vi "MapScriptActor.vi"(8 "error in (no error)":errorcluster) -> (0 "error out":errorcluster)   [LabVIEW 2017]
doc: "Use this template to build a VI to use as a subVI."
uses:
  MapScriptMeasurementStateMachineEnum.ctl
  Spectrometer Utilities/SpectrometerControllerEnum.ctl
  Spectrometer Utilities/SpectrometerCallbackdataEvent.ctl
  Microscope/MicroscopeControllerCluster.ctl
  <vilib>/vision/Image Controls.llb/IMAQ Image.ctl
  Microscope/MicroscopeControllerEnum.ctl
  Database/DatabaseContollerGFVenum.ctl
  MapScriptGFVEnum.ctl
  Spectrometer Utilities/SpectrometerData.ctl
  AEROTECstageAPI/StageEnum.ctl
  MapScriptDataGFV.ctl
  SpectroMeasurementCtrlEnum.ctl
panel:
  in  "Reset Measurement":bool
  in  "CaptureMicroscopeImageButton":bool
  out "User Picture":T1(plugin-control)
  in  "Add/Remove User 2":bool
  in  "Sample Type":u16(ring) caption="Combo Box" items=["Solid", "Liquid"]
  out "Experiment No.":i32 caption="String"
  in  "Experiment Title":string caption="String"
  out "Measurement State":T2
  out "Measurement points left in queue":i32
  out "Number of Points Selected":i32
  in  "abort":bool
  out "Measurement\nCompleted\nSuccessfully":bool
  out "Measurement\nIn\nProgress":bool
  in  "Stop":bool
  in  "Run":bool
  # "Map script"
  # "Total Measurment Time Estimate"
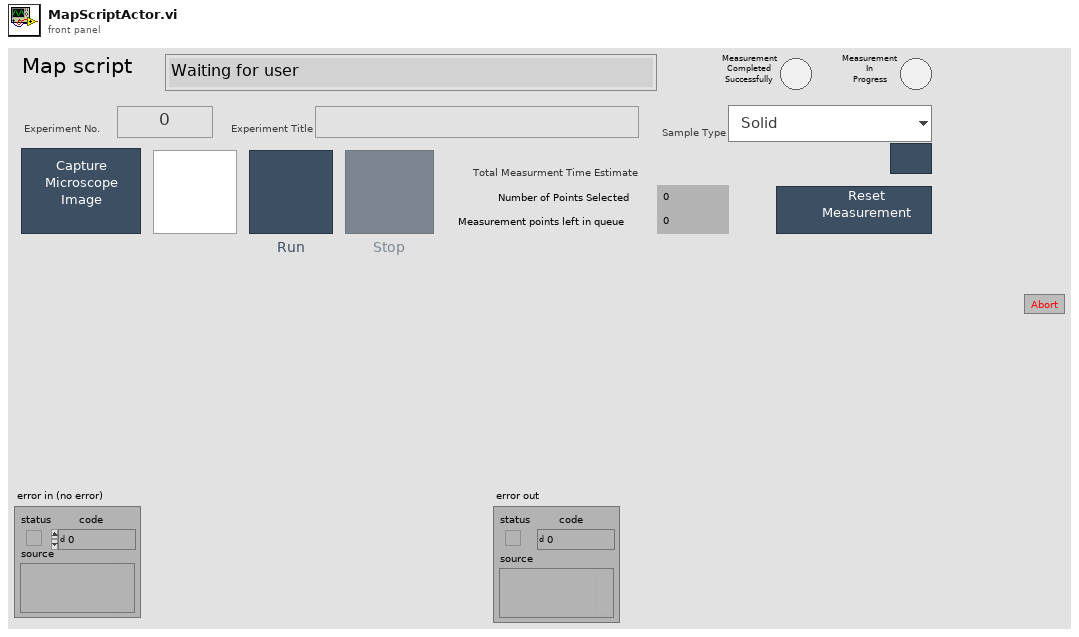
[diagram p1: front panel]
types:
  T1 = typedef "IMAQ Image.ctl" = refnum<image>
  T2 = typedef "MapScriptMeasurementStateMachineEnum.ctl" = enum16{"Waiting for user", "Moving the stage", "Verifying stage moved Successfully", "Running Raman measurement", "Waiting for measurement to finish", "Updating database with results"}
  T3 = typedef "MapScriptGFVEnum.ctl" = enum16{"GetAllData!", "InsertCoordData!", "InsertExperimentTitle", "Init!", "Stop!", "Start!", "GetMapScriptActorViRef", "InsertExperimentNumber", "InsertSampleType", "InsertMicroscopeImage"}
  T4 = typedef "DatabaseContollerGFVenum.ctl" = enum16{"Init and Open Database!", "GetNewMeas_dataIndex", "UpdateWithSpectrometerData", "UpdateWithMicroscopeData", "UpdateWithMapScriptData", "UpdateWithmainUIData", "Get Objective Microns/Pixels", "Get User Name!", "Get Active Users Names!", "Get User Picture!", "Get User Phone Number!", "Get Setup Names!", "Get Active Microscope Objectives!", "Get Experiment Number!", "Get Sample Types!", "Write meas_conf Table", "Write meas_data Table", "GetListOfIndices", "Get Objective Index"}
  T5 = cluster{"Stop":bool, "Point":cluster{"X":sgl, "Y":sgl}, "PointIndex":i32}
  T6 = typedef "MicroscopeControllerEnum.ctl" = enum16{"GetAllData!", "Init!", "Start!", "Stop!", "GetMicroscopeVIRef", "CalculateRelPointForStagemicrons", "InsertCallbackEvent!", "InsertLaserPoint!", "InsertMapPoints!", "InsertMicroscopeImageRef!", "GetMicroscopeImageRef", "InsertObjectiveIndex!"}
  T7 = typedef "SpectrometerControllerEnum.ctl" = enum16{"Init!", "Start!", "Stop!", "Start New Measurement!", "Update Current Measurement Data", "Set Current Measurement Ended Successfully", "Get Current Measurement Data!", "Get Current Measurement Ended Successfully", "GetSpectrometerVIRef!", "Insert Callback Event", "GetAllData!"}
  T8 = typedef "StageEnum.ctl" = enum16{"Get Current Pos!", "Move axis!", "Enable Stage!", "Stop Stage Controller!", "Set Default Speeds!", "Get Stage Parameters", "Start Stage Controller!", "Init", "Go Home!"}
  T9 = typedef "MapScriptDataGFV.ctl" = cluster{"idMeasConf":u32, "ExperimentTitle":string, "idsample_type":u32, "MicroscopeImage":string, "MeasPointNum":u32, "XCoorRequestedPixel":u32, "YCoorRequestedPixel":u32, "XCoorRequestedMicrons":dbl, "YCoorRequestedMicrons":dbl, "XCoorMeasuredMicrons":dbl, "YCoorMeasuredMicrons":dbl, "idMeasData":u32}
  T10 = typedef "MicroscopeControllerCluster.ctl" = cluster{"MapPointsArray":cluster{"X":i32, "Y":i32}[], "Laser Point Coor":cluster{"X":i32, "Y":i32}, "Microscope Image Ref":T1, "idObjectives":u32}
  T11 = typedef "SpectroMeasurementCtrlEnum.ctl" = enum16{"Init", "InsertMeasurementScript", "InsertSetupIndex", "InsertCurrentUserIndex", "GetAllData!"}
  T12 = typedef "SpectrometerData.ctl" = cluster{"Acquisition Time":dbl, "Range Begin":dbl, "Acquistion Time Unit":string, "Accumulations":i32, "Range End":dbl, "Range Unit":string, "Windows":i32, "Auto Focus":bool, "Auto Exposure":bool, "Spike Filter":string, "Delay Time":dbl, "Delay Time Unit":string, "Binning":i32, "Readout Mode":string, "DeNoise":bool, "ICS correction":bool, "Dark correction":bool, "Instrument Process":bool, "Instrument":string, "Detector":string, "Objective":string, "Grating":i32, "Grating Unit":string, "ND Filter":dbl, "ND Filter Unit":string, "Laser":dbl, "Laser Unit":string, "Slit":dbl, "Hole":dbl, "Acquired DateTime":string, "X axis":dbl[], "Y axis":dbl[]}
  T13 = enum8{"Enabled", "Disabled", "Disabled and Grayed Out"}
  T14 = typedef "SpectrometerCallbackdataEvent.ctl" = cluster{"MeasurementEndedSuccessfully?":bool, "Spectrometer Connected?":bool, "Measurement In Progress?":bool}
  T15 = typedef "Image Type" = u32
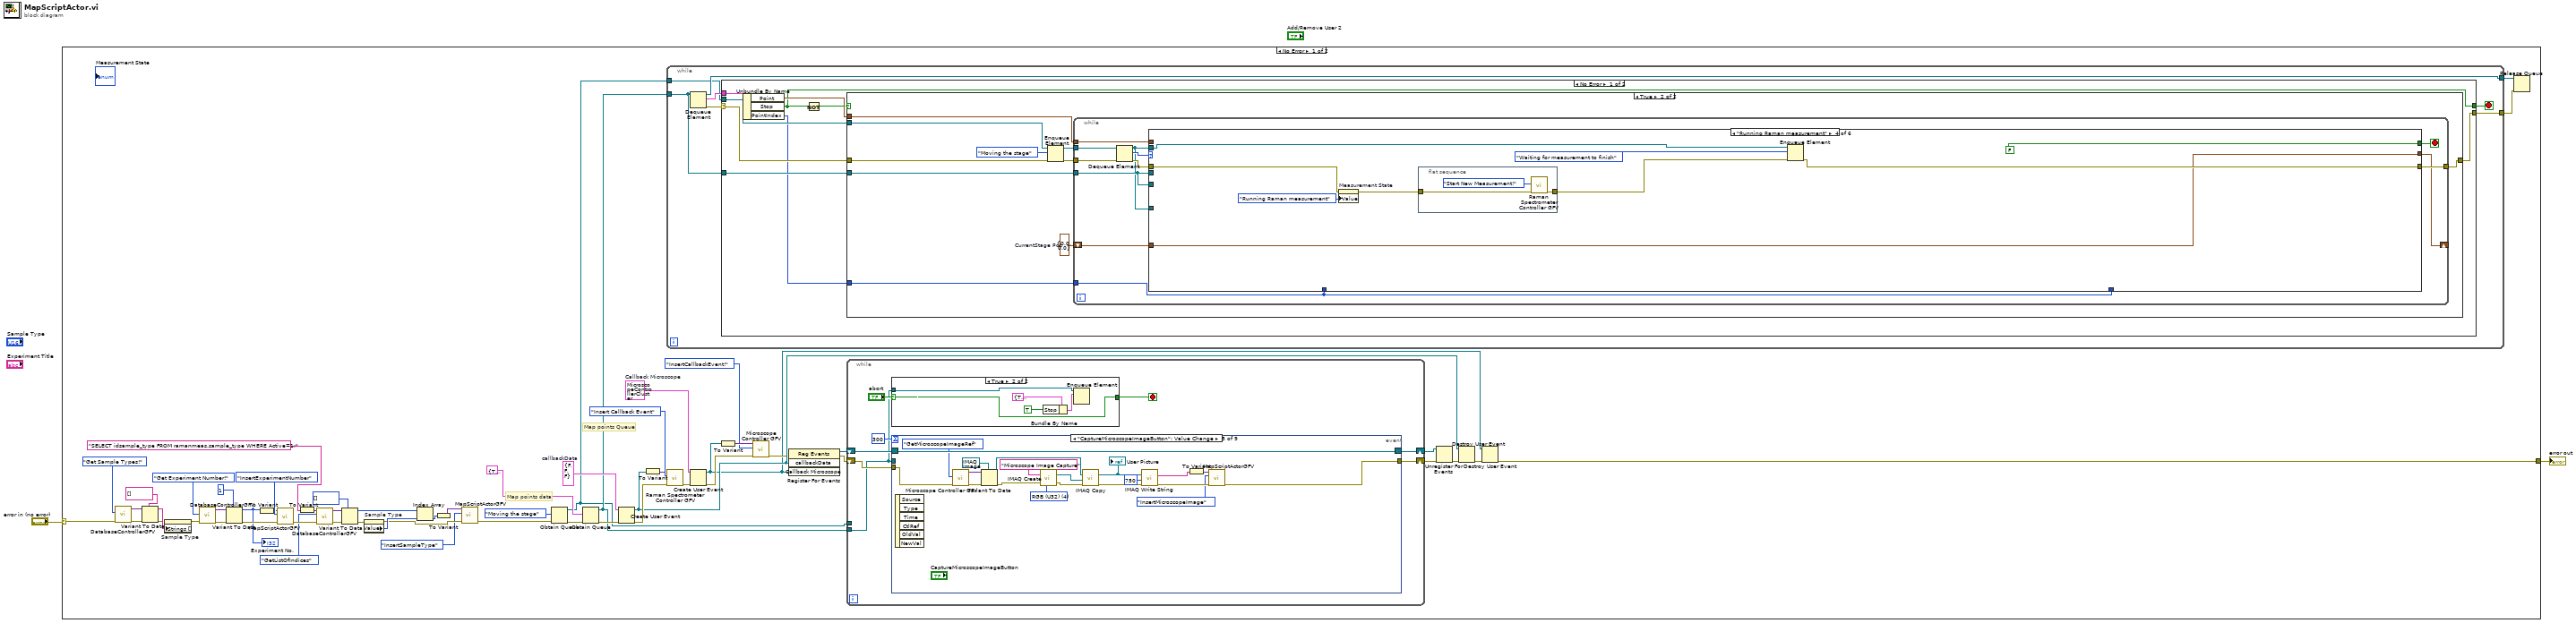
[diagram p0: block diagram]
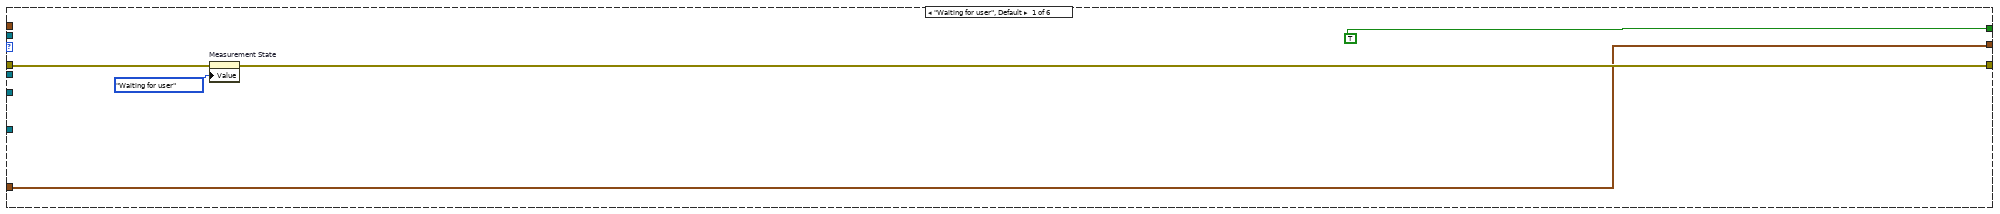
[diagram p3: hidden frame]
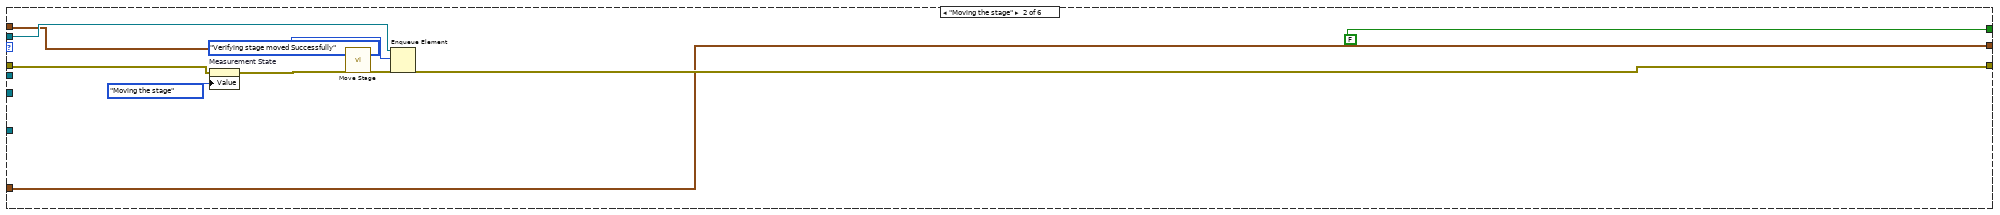
[diagram p4: hidden frame]
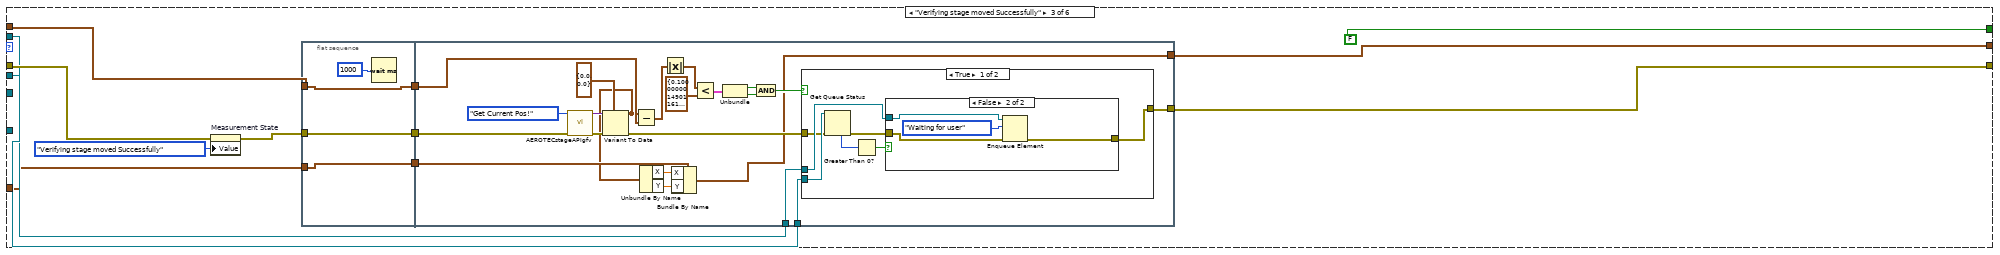
[diagram p5: hidden frame]
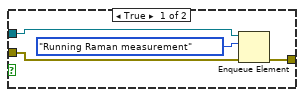
[diagram p6: hidden frame]
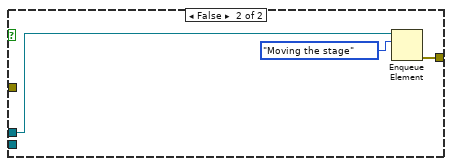
[diagram p7: hidden frame]
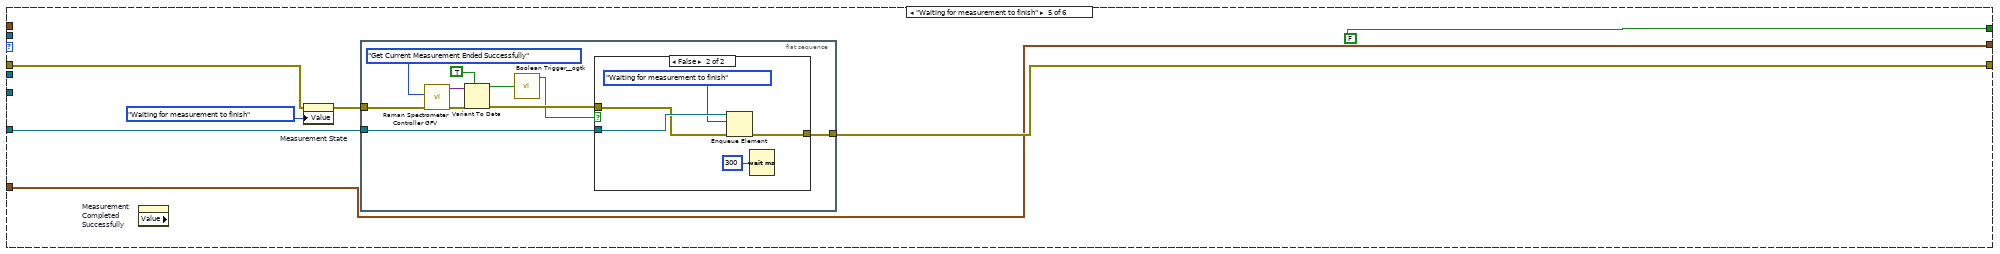
[diagram p8: hidden frame]
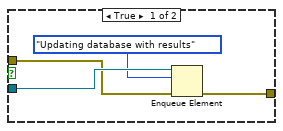
[diagram p9: hidden frame]
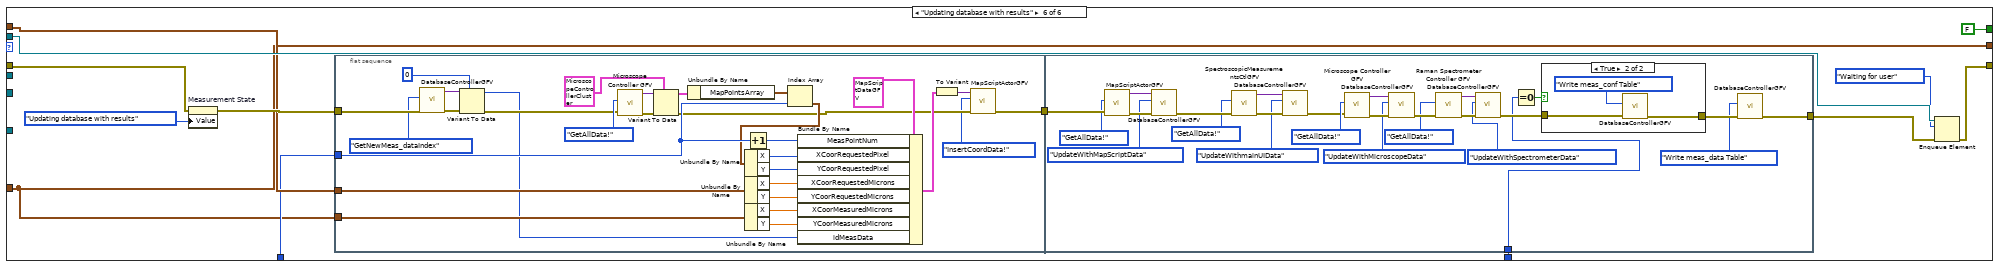
[diagram p10: hidden frame]
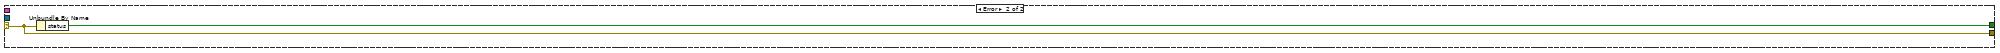
[diagram p12: hidden frame]
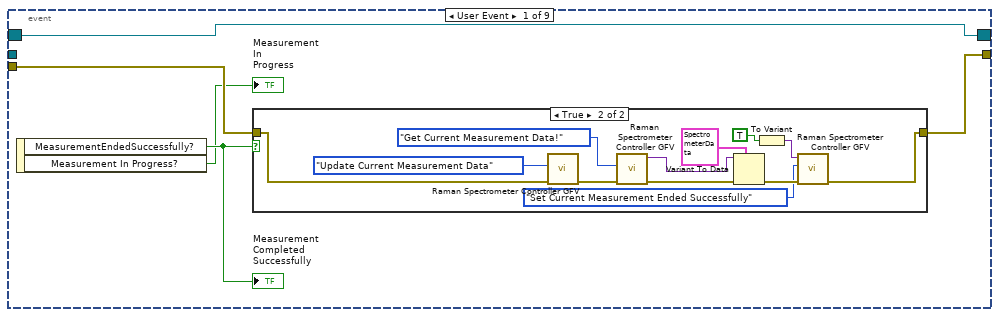
[diagram p14: hidden frame]
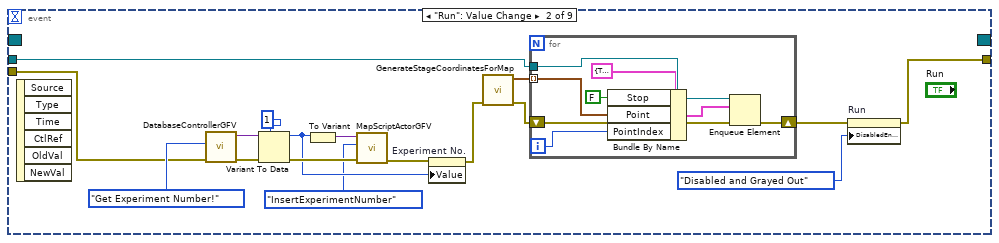
[diagram p16: hidden frame]
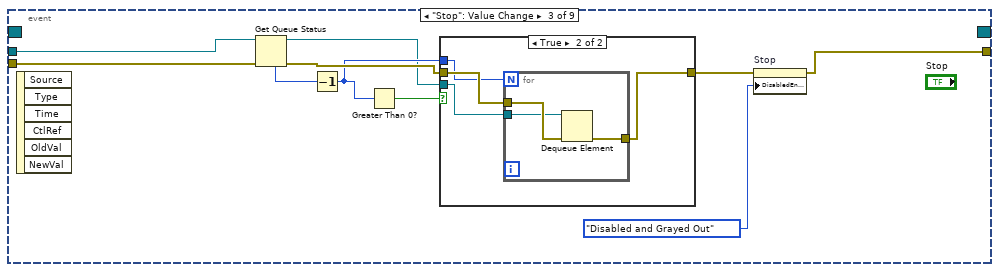
[diagram p17: hidden frame]
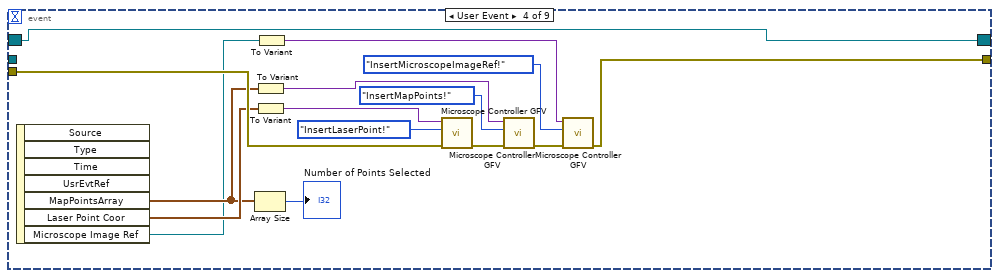
[diagram p19: hidden frame]
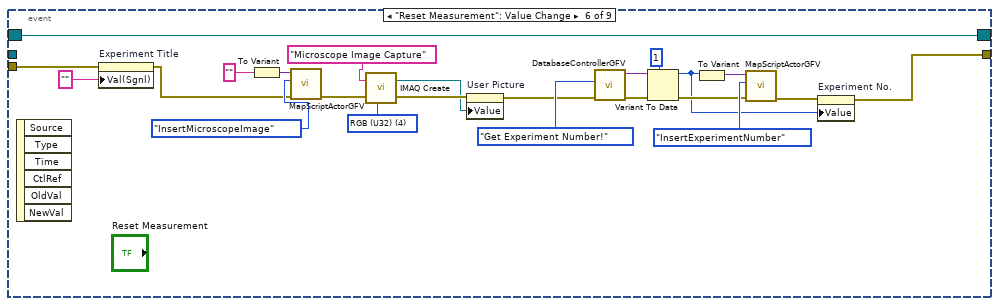
[diagram p20: hidden frame]
diagram:
  n1 = case shown="No Error" "error in (no error)" {
    selector: "error in (no error)" -> [w22 w456]
    tunnel: [w38 w456] -> w1
    frame No Error {
      w50 = T10 {"MapPointsArray"=[], "Laser Point Coor"={"X"=0, "Y"=0}, "Microscope Image Ref"=refnum, "idObjectives"=0}  # Callback Microscope
      w59 = T14 {"MeasurementEndedSuccessfully?"=FALSE, "Spectrometer Connected?"=FALSE, "Measurement In Progress?"=FALSE}  # callbackData
      # "Map points data"
      # "Map points Queue"
      n2 = call "DatabaseControllerGFV.vi"("error in (no error)"=w22, "Enum"=DatabaseContollerGFVenum."Get Sample Types!") -> ("error out"=w29:errorcluster, "Data Out"=w28:variant)  [unwired: 8 in]
      n3 = Variant To Data(error in=w29, type=string[] [] ("Strings []"), Variant=w28) -> (data=w25:string[], error out=w23:errorcluster)
      n4 = property on="Sample Type" class="Ring (strict)"(error in=w23, "Strings []"=w25) -> (error out=w24:errorcluster)  [unwired: 1 in, 1 out]
      n5 = call "DatabaseControllerGFV.vi"("error in (no error)"=w24, "Enum"=DatabaseContollerGFVenum."Get Experiment Number!") -> ("error out"=w31:errorcluster, "Data Out"=w32:variant)  [unwired: 8 in]
      n6 = Variant To Data(error in=w31, type=1, Variant=w32) -> (data=w18:i32, error out=w21:errorcluster)
      "Experiment No." <- w18
      n7 = To Variant(anything=w18) -> (Variant=w19:variant)
      n8 = call "MapScriptActorGFV.vi"("error in (no error)"=w21, "MapScriptEnum"=MapScriptGFVEnum."InsertExperimentNumber", "Data in"=w19) -> ("error out"=w17:errorcluster)  [unwired: 7 in, 1 out]
      n9 = To Variant(anything="SELECT idsample_type FROM ramanmeas.sample_type WHERE Active=1;") -> (Variant=w16:variant)
      n10 = call "DatabaseControllerGFV.vi"("error in (no error)"=w17, "Enum"=DatabaseContollerGFVenum."GetListOfIndices", "Data in"=w16) -> ("error out"=w13:errorcluster, "Data Out"=w12:variant)  [unwired: 7 in]
      n11 = Variant To Data(error in=w13, type=i32[] [], Variant=w12) -> (data=w10:i32[], error out=w9:errorcluster)
      n12 = property on="Sample Type" class="Ring (strict)"(error in=w9) -> (error out=w7:errorcluster, "Value"=w8:u16)  [unwired: 1 in, 1 out]
      n13 = Index Array(array=w10, index=w8) -> (element=w4:i32)
      n14 = To Variant(anything=w4) -> (Variant=w3:variant)
      n15 = call "MapScriptActorGFV.vi"("error in (no error)"=w7, "MapScriptEnum"=MapScriptGFVEnum."InsertSampleType", "Data in"=w3) -> ("error out"=w6:errorcluster)  [unwired: 7 in, 1 out]
      n16 = Obtain Queue(element data type=MapScriptMeasurementStateMachineEnum."Moving the stage" ("element"), error in (no error)=w6) -> (queue out=w35:refnum<queue>, error out=w36:errorcluster)  [unwired: 3 in, 1 out]
      n17 = Obtain Queue(element data type=T5 {"Stop"=TRUE, "Point"={"X"=0.0, "Y"=0.0}, "PointIndex"=0}, error in (no error)=w36) -> (queue out=w41:refnum<queue>, error out=w42:errorcluster)  [unwired: 3 in, 1 out]
      n18 = Create User Event(user event datatype=w59, error in=w42) -> (user event=w52:refnum<user-event>, error out=w58:errorcluster)
      n19 = To Variant(anything=w52) -> (Variant=w57:variant)
      n20 = while {
        tunnel: w41 -> [w61]
        tunnel: [w65] -> w40
        tunnel: [w64] -> w39
        tunnel: w35 -> [w62]
        stop <- w63 stop-if-true
        n21 = Dequeue Element(queue=w61) -> (queue out=w65:refnum<queue>, element=w66:T5, error out=w67:errorcluster)  [unwired: 2 in, 1 out]
        n22 = case shown="No Error" w67 {
          selector: w67 -> [w72 w284]
          tunnel: w66 -> [w76 _]
          tunnel: [w71 w284] -> w64
          tunnel: [w73 w283] -> w63
          tunnel: w62 -> [w70 _]
          tunnel: w61 -> [w69 _]
          frame No Error {
            n23 = Unbundle By Name(w76) -> ("Point"=w75:cluster{"X":sgl, "Y":sgl}, "Stop"=w73:bool, "PointIndex"=w68:i32)
            n24 = Not(x=w73) -> (.not. x?=w74:bool)
            n25 = case shown="True" w74 {
              tunnel: w75 -> [_ w87]
              tunnel: w72 -> [w77 w84]
              tunnel: [w77 w82] -> w71
              tunnel: w70 -> [_ w86]
              tunnel: w69 -> [_ w80]
              tunnel: w68 -> [_ w78]
              frame False {
              }
              frame True {
                w79 = cluster{"X":sgl, "Y":sgl} {"X"=0.0, "Y"=0.0}  # CurrentStage Pos
                n26 = Enqueue Element(queue=w86, element=MapScriptMeasurementStateMachineEnum."Moving the stage", error in (no error)=w84) -> (queue out=w85:refnum<queue>, error out=w83:errorcluster)  [unwired: 1 in, 1 out]
                n27 = while {
                  tunnel: w85 -> [w99]
                  tunnel: w83 -> [w98]
                  tunnel: w87 -> [w95]
                  tunnel: [w91] -> w82
                  tunnel: w80 -> [w93]
                  shift-right: [w90] -> _
                  shift-left: w79 -> [w88]
                  tunnel: w78 -> [w89]
                  stop <- w96 stop-if-true
                  n28 = Dequeue Element(queue=w99, error in (no error)=w98) -> (queue out=w92:refnum<queue>, element=w94:T2, error out=w97:errorcluster)  [unwired: 1 in, 1 out]
                  n29 = case shown="\"Running Raman measurement\"" w94 {
                    tunnel: w97 -> [w102 w113 w126 w179 w190 w221]
                    tunnel: [TRUE FALSE FALSE FALSE FALSE FALSE] -> w96
                    tunnel: w95 -> [_ w108 w123 _ _ w213]
                    tunnel: w92 -> [_ w112 w120 w177 _ w218]
                    tunnel: w93 -> [_ _ _ _ _ _]
                    tunnel: w93 -> [_ _ w122 _ _ _]
                    tunnel: [w101 w106 w121 w175 w186 w215] -> w91
                    tunnel: w92 -> [_ _ _ _ w187 _]
                    tunnel: [w100 w105 w117 w172 w184 w211] -> w90
                    tunnel: w88 -> [w100 w105 w116 w172 w184 w211]
                    tunnel: w89 -> [_ _ _ _ _ w212]
                    tunnel: w89 -> [_ _ _ _ _ w210]
                    frame "Waiting for user", Default {
                      n30 = property on="Measurement State" class="Enum (strict)"(error in=w102, "Value"=MapScriptMeasurementStateMachineEnum."Waiting for user" ("element")) -> (error out=w101:errorcluster)  [unwired: 1 in, 1 out]
                    }
                    frame "Moving the stage" {
                      n31 = property on="Measurement State" class="Enum (strict)"(error in=w113, "Value"=MapScriptMeasurementStateMachineEnum."Moving the stage" ("element")) -> (error out=w109:errorcluster)  [unwired: 1 in, 1 out]
                      n32 = call "Move Stage.vi"("error in (no error)"=w109, "Input Coor"=w108) -> ("error out"=w107:errorcluster)  [unwired: 9 in]
                      n33 = Enqueue Element(queue=w112, element=MapScriptMeasurementStateMachineEnum."Verifying stage moved Successfully", error in (no error)=w107) -> (error out=w106:errorcluster)  [unwired: 1 in, 2 out]
                    }
                    frame "Verifying stage moved Successfully" {
                      n34 = property on="Measurement State" class="Enum (strict)"(error in=w126, "Value"=MapScriptMeasurementStateMachineEnum."Verifying stage moved Successfully" ("element")) -> (error out=w125:errorcluster)  [unwired: 1 in, 1 out]
                      n35 = flat-sequence {
                        tunnel: w123 -> [w130]
                        tunnel: w125 -> [w131]
                        tunnel: [w131] -> w119
                        tunnel: [w130] -> w118
                        tunnel: w116 -> [w128]
                        tunnel: [w128] -> w115
                        tunnel: w120 -> [w140]
                        tunnel: w122 -> [w139]
                        tunnel: [w138] -> w121
                        tunnel: w119 -> [w149]
                        tunnel: w118 -> [w148]
                        tunnel: [w135] -> w117
                        tunnel: w115 -> [w136]
                        frame #0 {
                          n36 = Wait (ms)(milliseconds to wait=u32 1000) -> ()  [unwired: 1 out]
                        }
                        frame #1 {
                          n37 = call "AEROTECstageAPIgfv.vi"("error in (no error)"=w149, "StageContrlEnum"=StageEnum."Get Current Pos!") -> ("error out"=w150:errorcluster, "Data Out"=w152:variant)  [unwired: 8 in]
                          n38 = Variant To Data(error in=w150, type=cluster{"X":sgl, "Y":sgl} {"X"=0.0, "Y"=0.0}, Variant=w152) -> (data=w134:cluster{"X":sgl, "Y":sgl}, error out=w137:errorcluster)
                          n39 = Subtract(x=w134, y=w148) -> (x-y=w147:cluster{"X":sgl, "Y":sgl})
                          n40 = Unbundle By Name(w134) -> ("X"=w133:sgl, "Y"=w132:sgl)
                          n41 = Absolute Value(x=w147) -> (abs(x)=w146:cluster{"X":sgl, "Y":sgl})
                          n42 = Bundle By Name(cluster=w136, "X"=w133, "Y"=w132) -> (w135:cluster{"X":sgl, "Y":sgl})
                          n43 = Less?(x=w146, y=cluster{"X":sgl, "Y":sgl} {"X"=0.1, "Y"=0.1}) -> (x < y?=w144:cluster{"X":bool, "Y":bool})
                          n44 = Unbundle(w144) -> ("X"=w143:bool, "Y"=w142:bool)
                          n45 = And(x=w143, y=w142) -> (x .and. y?=w141:bool)
                          n46 = case shown="True" w141 {
                            tunnel: w140 -> [w157 w171]
                            tunnel: w139 -> [w156 _]
                            tunnel: [w155 w170] -> w138
                            tunnel: w137 -> [w154 _]
                            frame True {
                              n47 = Get Queue Status(queue=w156, error in (no error)=w154) -> (error out=w158:errorcluster, # elements in queue=w159:i32)  [unwired: 1 in, 6 out]
                              n48 = Greater Than 0?(x=w159) -> (x > 0?=w160:bool)
                              n49 = case shown="False" w160 {
                                tunnel: [w164 w168] -> w155
                                tunnel: w157 -> [w163 w167]
                                tunnel: w158 -> [w161 w165]
                                frame True {
                                n50 = Enqueue Element(queue=w163, element=MapScriptMeasurementStateMachineEnum."Running Raman measurement", error in (no error)=w161) -> (error out=w164:errorcluster)  [unwired: 1 in, 2 out]
                                }
                                frame False {
                                n51 = Enqueue Element(queue=w167, element=MapScriptMeasurementStateMachineEnum."Waiting for user", error in (no error)=w165) -> (error out=w168:errorcluster)  [unwired: 1 in, 2 out]
                                }
                              }
                            }
                            frame False {
                              n52 = Enqueue Element(queue=w171, element=MapScriptMeasurementStateMachineEnum."Moving the stage") -> (error out=w170:errorcluster)  [unwired: 2 in, 2 out]
                            }
                          }
                        }
                      }
                    }
                    frame "Running Raman measurement" {
                      n53 = property on="Measurement State" class="Enum (strict)"(error in=w179, "Value"=MapScriptMeasurementStateMachineEnum."Running Raman measurement" ("element")) -> (error out=w178:errorcluster)  [unwired: 1 in, 1 out]
                      n54 = flat-sequence {
                        tunnel: w178 -> [w182]
                        tunnel: [w181] -> w174
                        frame #0 {
                          n55 = call "Raman Spectrometer Controller GFV.vi"("SpectrometerEnum"=SpectrometerControllerEnum."Start New Measurement!", "error in (no error)"=w182) -> ("error out"=w181:errorcluster)  [unwired: 7 in, 1 out]
                        }
                      }
                      n56 = Enqueue Element(queue=w177, element=MapScriptMeasurementStateMachineEnum."Waiting for measurement to finish", error in (no error)=w174) -> (error out=w175:errorcluster)  [unwired: 1 in, 2 out]
                    }
                    frame "Waiting for measurement to finish" {
                      n57 = property on="Measurement\nCompleted\nSuccessfully" class="Bool (strict)" props=["Value"]() -> ()  [unwired: 2 in, 3 out]
                      n58 = property on="Measurement State" class="Enum (strict)"(error in=w190, "Value"=MapScriptMeasurementStateMachineEnum."Waiting for measurement to finish" ("element")) -> (error out=w189:errorcluster)  [unwired: 1 in, 1 out]
                      n59 = flat-sequence {
                        tunnel: w189 -> [w198]
                        tunnel: w187 -> [w200]
                        tunnel: [w199] -> w186
                        frame #0 {
                          n60 = call "Raman Spectrometer Controller GFV.vi"("SpectrometerEnum"=SpectrometerControllerEnum."Get Current Measurement Ended Successfully", "error in (no error)"=w198) -> ("Data Out"=w195:variant, "error out"=w196:errorcluster)  [unwired: 7 in]
                          n61 = Variant To Data(error in=w196, type=TRUE, Variant=w195) -> (data=w192:bool, error out=w193:errorcluster)
                          n62 = call <userlib>:"Boolean Trigger__ogtk.vi"("Boolean Input"=w192) -> ("Rising Edge"=w191:bool)  [unwired: 1 in, 1 out]
                          n63 = case shown="False" w191 {
                            tunnel: w200 -> [w204 w209]
                            tunnel: [w203 w208] -> w199
                            tunnel: w193 -> [w201 w206]
                            frame True {
                              n64 = Enqueue Element(queue=w204, element=MapScriptMeasurementStateMachineEnum."Updating database with results", error in (no error)=w201) -> (error out=w203:errorcluster)  [unwired: 1 in, 2 out]
                            }
                            frame False {
                              n65 = Enqueue Element(queue=w209, element=MapScriptMeasurementStateMachineEnum."Waiting for measurement to finish", error in (no error)=w206) -> (error out=w208:errorcluster)  [unwired: 1 in, 2 out]
                              n66 = Wait (ms)(milliseconds to wait=u32 300) -> ()  [unwired: 1 out]
                            }
                          }
                        }
                      }
                    }
                    frame "Updating database with results" {
                      n67 = property on="Measurement State" class="Enum (strict)"(error in=w221, "Value"=MapScriptMeasurementStateMachineEnum."Updating database with results" ("element")) -> (error out=w220:errorcluster)  [unwired: 1 in, 1 out]
                      n68 = flat-sequence {
                        tunnel: w220 -> [w229]
                        tunnel: [w231] -> w214
                        tunnel: w213 -> [w240]
                        tunnel: w211 -> [w243]
                        tunnel: w212 -> [w244]
                        tunnel: [w254] -> w219
                        tunnel: w214 -> [w278]
                        tunnel: w210 -> [w256]
                        frame #0 {
                          n69 = call "DatabaseControllerGFV.vi"("error in (no error)"=w229, "Enum"=DatabaseContollerGFVenum."GetNewMeas_dataIndex") -> ("error out"=w228:errorcluster, "Data Out"=w225:variant)  [unwired: 8 in]
                          n70 = Variant To Data(error in=w228, type=0, Variant=w225) -> (data=w223:i32, error out=w227:errorcluster)
                          n71 = call "Microscope Controller GFV.vi"("error in (no error)"=w227, "MicroscopeEnum"=MicroscopeControllerEnum."GetAllData!") -> ("error out"=w251:errorcluster, "Data Out"=w250:variant)  [unwired: 8 in]
                          n72 = Variant To Data(error in=w251, type=T10 {"MapPointsArray"=[], "Laser Point Coor"={"X"=0, "Y"=0}, "Microscope Image Ref"=refnum, "idObjectives"=0}, Variant=w250) -> (data=w248:T10, error out=w232:errorcluster)
                          n73 = Unbundle By Name(w248) -> ("MapPointsArray"=w247:cluster{"X":i32, "Y":i32}[])
                          n74 = Unbundle By Name(w240) -> ("X"=w239:sgl, "Y"=w238:sgl)
                          n75 = Unbundle By Name(w243) -> ("X"=w242:sgl, "Y"=w241:sgl)
                          n76 = Increment(x=w244) -> (x+1=w245:i32)
                          n77 = Index Array(array=w247, index=w244) -> (element=w237:cluster{"X":i32, "Y":i32})
                          n78 = Unbundle By Name(w237) -> ("X"=w236:i32, "Y"=w235:i32)
                          n79 = Bundle By Name(cluster=T9 {"idMeasConf"=0, "ExperimentTitle"="", "idsample_type"=0, "MicroscopeImage"="", "MeasPointNum"=0, "XCoorRequestedPixel"=0, "YCoorRequestedPixel"=0, "XCoorRequestedMicrons"=0.0, "YCoorRequestedMicrons"=0.0, "XCoorMeasuredMicrons"=0.0, "YCoorMeasuredMicrons"=0.0, "idMeasData"=0}, "MeasPointNum"=w245, "XCoorRequestedPixel"=w236, "YCoorRequestedPixel"=w235, "XCoorRequestedMicrons"=w239, "YCoorRequestedMicrons"=w238, "XCoorMeasuredMicrons"=w242, "YCoorMeasuredMicrons"=w241, "idMeasData"=w223) -> (w233:T9)
                          n80 = To Variant(anything=w233) -> (Variant=w234:variant)
                          n81 = call "MapScriptActorGFV.vi"("error in (no error)"=w232, "MapScriptEnum"=MapScriptGFVEnum."InsertCoordData!", "Data in"=w234) -> ("error out"=w231:errorcluster)  [unwired: 7 in, 1 out]
                        }
                        frame #1 {
                          n82 = call "MapScriptActorGFV.vi"("error in (no error)"=w278, "MapScriptEnum"=MapScriptGFVEnum."GetAllData!") -> ("error out"=w277:errorcluster, "Data Out"=w275:variant)  [unwired: 8 in]
                          n83 = call "DatabaseControllerGFV.vi"("error in (no error)"=w277, "Enum"=DatabaseContollerGFVenum."UpdateWithMapScriptData", "Data in"=w275) -> ("error out"=w273:errorcluster)  [unwired: 7 in, 1 out]
                          n84 = call "SpectroscopicMeasurementsCtlGFV.vi"("error in (no error)"=w273, "Enum"=SpectroMeasurementCtrlEnum."GetAllData!") -> ("error out"=w271:errorcluster, "Data Out"=w269:variant)  [unwired: 8 in]
                          n85 = call "DatabaseControllerGFV.vi"("error in (no error)"=w271, "Enum"=DatabaseContollerGFVenum."UpdateWithmainUIData", "Data in"=w269) -> ("error out"=w267:errorcluster)  [unwired: 7 in, 1 out]
                          n86 = call "Microscope Controller GFV.vi"("error in (no error)"=w267, "MicroscopeEnum"=MicroscopeControllerEnum."GetAllData!") -> ("error out"=w266:errorcluster, "Data Out"=w265:variant)  [unwired: 8 in]
                          n87 = call "DatabaseControllerGFV.vi"("error in (no error)"=w266, "Enum"=DatabaseContollerGFVenum."UpdateWithMicroscopeData", "Data in"=w265) -> ("error out"=w263:errorcluster)  [unwired: 7 in, 1 out]
                          n88 = call "Raman Spectrometer Controller GFV.vi"("SpectrometerEnum"=SpectrometerControllerEnum."GetAllData!", "error in (no error)"=w263) -> ("Data Out"=w260:variant, "error out"=w261:errorcluster)  [unwired: 7 in]
                          n89 = call "DatabaseControllerGFV.vi"("error in (no error)"=w261, "Enum"=DatabaseContollerGFVenum."UpdateWithSpectrometerData", "Data in"=w260) -> ("error out"=w258:errorcluster)  [unwired: 7 in, 1 out]
                          n90 = Equal To 0?(x=w256) -> (x = 0?=w257:bool)
                          n91 = case shown="True" w257 {
                            tunnel: w258 -> [w279 w282]
                            tunnel: [w279 w281] -> w255
                            frame False {
                            }
                            frame True {
                              n92 = call "DatabaseControllerGFV.vi"("error in (no error)"=w282, "Enum"=DatabaseContollerGFVenum."Write meas_conf Table") -> ("error out"=w281:errorcluster)  [unwired: 8 in, 1 out]
                            }
                          }
                          n93 = call "DatabaseControllerGFV.vi"("error in (no error)"=w255, "Enum"=DatabaseContollerGFVenum."Write meas_data Table") -> ("error out"=w254:errorcluster)  [unwired: 8 in, 1 out]
                        }
                      }
                      n94 = Enqueue Element(queue=w218, element=MapScriptMeasurementStateMachineEnum."Waiting for user", error in (no error)=w219) -> (error out=w215:errorcluster)  [unwired: 1 in, 2 out]
                    }
                  }
                }
              }
            }
          }
          frame Error {
            n95 = Unbundle By Name(w284) -> ("status"=w283:bool)
          }
        }
      }
      n96 = call "Raman Spectrometer Controller GFV.vi"("Data in"=w57, "SpectrometerEnum"=SpectrometerControllerEnum."Insert Callback Event", "error in (no error)"=w58) -> ("error out"=w47:errorcluster)  [unwired: 6 in, 1 out]
      n97 = Create User Event(user event datatype=w50, error in=w47) -> (user event=w43:refnum<user-event>, error out=w48:errorcluster)
      n98 = To Variant(anything=w43) -> (Variant=w49:variant)
      n99 = call "Microscope Controller GFV.vi"("error in (no error)"=w48, "MicroscopeEnum"=MicroscopeControllerEnum."InsertCallbackEvent!", "Data in"=w49) -> ("error out"=w46:errorcluster)  [unwired: 7 in, 1 out]
      n100 = register-events(error in=w46, w52, w43) -> (reference out=w55:refnum<event-registration>, error out=w56:errorcluster)  [unwired: 1 in]
      n101 = while {
        shift-right: [w285] -> w54
        shift-left: w56 -> [w289]
        shift-right: [w290] -> w53
        shift-left: w55 -> [w292]
        tunnel: w41 -> [w286]
        tunnel: w35 -> [_]
        stop <- w287 stop-if-true
        n102 = case shown="True" "abort" {
          selector: "abort" -> [w293 w295]
          tunnel: w286 -> [_ w296]
          tunnel: [w293 w295] -> w287
          frame False {
          }
          frame True {
            n103 = Bundle By Name(cluster=T5 {"Stop"=TRUE, "Point"={"X"=0.0, "Y"=0.0}, "PointIndex"=0}, "Stop"=TRUE) -> (w298:T5)
            n104 = Enqueue Element(queue=w296, element=w298) -> ()  [unwired: 2 in, 3 out]
          }
        }
        n105 = event shown="[4] \"CaptureMicroscopeImageButton\": Value Change" {
          selector: w292 -> [w301 _ _ w373 w394 w416 w432 w438 w445]
          dyn-events: [w301 _ _ w373 w394 w416 w432 w438 w445] -> w290
          timeout: 300 -> [_ _ _ _ _ _ _ _ _]
          tunnel: w289 -> [w303 w318 w350 w372 w393 w417 w419 w437 w441]
          tunnel: [w302 w329 w343 w360 w375 w400 w418 w434 w440] -> w285
          tunnel: w286 -> [_ w333 w351 _ _ _ _ _ w444]
          event User Event {
            n106 = event-data() -> ("MeasurementEndedSuccessfully?"=w300:bool, "Measurement In Progress?"=→"Measurement\nIn\nProgress":bool)  [unwired: 1 in]
            "Measurement\nCompleted\nSuccessfully" <- w300
            n107 = case shown="True" w300 {
              tunnel: w303 -> [w304 w310]
              tunnel: [w304 w308] -> w302
              frame False {
              }
              frame True {
                n108 = call "Raman Spectrometer Controller GFV.vi"("SpectrometerEnum"=SpectrometerControllerEnum."Update Current Measurement Data", "error in (no error)"=w310) -> ("error out"=w314:errorcluster)  [unwired: 7 in, 1 out]
                n109 = call "Raman Spectrometer Controller GFV.vi"("SpectrometerEnum"=SpectrometerControllerEnum."Get Current Measurement Data!", "error in (no error)"=w314) -> ("Data Out"=w316:variant, "error out"=w315:errorcluster)  [unwired: 7 in]
                n110 = Variant To Data(error in=w315, type=T12 {"Acquisition Time"=0.0, "Range Begin"=0.0, "Acquistion Time Unit"="", "Accumulations"=0, "Range End"=0.0, "Range Unit"="", "Windows"=0, "Auto Focus"=FALSE, "Auto Exposure"=FALSE, "Spike Filter"="", "Delay Time"=0.0, "Delay Time Unit"="", "Binning"=0, "Readout Mode"="", "DeNoise"=FALSE, "ICS correction"=FALSE, "Dark correction"=FALSE, "Instrument Process"=FALSE, "Instrument"="", "Detector"="", "Objective"="", "Grating"=0, "Grating Unit"="", "ND Filter"=0.0, "ND Filter Unit"="", "Laser"=0.0, "Laser Unit"="", "Slit"=0.0, "Hole"=0.0, "Acquired DateTime"="", "X axis"=[], "Y axis"=[]} ("Spectrometer Data"), Variant=w316) -> (error out=w309:errorcluster)  [unwired: 1 out]
                n111 = To Variant(anything=TRUE) -> (Variant=w306:variant)
                n112 = call "Raman Spectrometer Controller GFV.vi"("Data in"=w306, "SpectrometerEnum"=SpectrometerControllerEnum."Set Current Measurement Ended Successfully", "error in (no error)"=w309) -> ("error out"=w308:errorcluster)  [unwired: 6 in, 1 out]
              }
            }
          }
          event "Run": Value Change {
            n113 = event-data() -> ()  [unwired: 1 in, 6 out]
            n114 = call "DatabaseControllerGFV.vi"("error in (no error)"=w318, "Enum"=DatabaseContollerGFVenum."Get Experiment Number!") -> ("error out"=w325:errorcluster, "Data Out"=w324:variant)  [unwired: 8 in]
            n115 = Variant To Data(error in=w325, type=1, Variant=w324) -> (data=w323:i32, error out=w326:errorcluster)
            n116 = To Variant(anything=w323) -> (Variant=w327:variant)
            n117 = call "MapScriptActorGFV.vi"("error in (no error)"=w326, "MapScriptEnum"=MapScriptGFVEnum."InsertExperimentNumber", "Data in"=w327) -> ("error out"=w322:errorcluster)  [unwired: 7 in, 1 out]
            n118 = property on="Experiment No." class="DigNum (strict)"(error in=w322, "Value"=w323) -> (error out=w317:errorcluster)  [unwired: 1 in, 1 out]
            n119 = call "GenerateStageCoordinatesForMap.vi"("error in (no error)"=w317) -> ("error out"=w332:errorcluster, "Stage Coordinates for Map"=w331:cluster{"X":sgl, "Y":sgl}[])  [unwired: 9 in]
            n120 = for {
              tunnel: w333 -> [w340]
              shift-right: [w339] -> w330
              shift-left: w332 -> [w341]
              tunnel: w331 -> [w337] mode=indexing
              i -> [w334]
              n121 = Bundle By Name(cluster=T5 {"Stop"=TRUE, "Point"={"X"=0.0, "Y"=0.0}, "PointIndex"=0}, "Stop"=FALSE, "Point"=w337, "PointIndex"=w334) -> (w336:T5)
              n122 = Enqueue Element(queue=w340, element=w336, error in (no error)=w341) -> (error out=w339:errorcluster)  [unwired: 1 in, 2 out]
            }
            n123 = property on="Run" class="Bool"(error in=w330, "DisabledEnum"=T13."Disabled and Grayed Out" ("Disabled")) -> (error out=w329:errorcluster)  [unwired: 1 in, 1 out]
          }
          event "Stop": Value Change {
            n124 = event-data() -> ()  [unwired: 1 in, 6 out]
            n125 = Get Queue Status(queue=w351, error in (no error)=w350) -> (queue out=w345:refnum<queue>, error out=w349:errorcluster, # elements in queue=w348:i32)  [unwired: 1 in, 5 out]
            n126 = Decrement(x=w348) -> (x-1=w346:i32)
            n127 = Greater Than 0?(x=w346) -> (x > 0?=w347:bool)
            n128 = case shown="True" w347 {
              tunnel: w349 -> [w352 w356]
              tunnel: w346 -> [_ w355]
              tunnel: w345 -> [_ w354]
              tunnel: [w352 w353] -> w342
              frame False {
              }
              frame True {
                n129 = for {
                  N: w355 -> [_]
                  tunnel: w356 -> [w359]
                  tunnel: w354 -> [w358]
                  tunnel: [w357] -> w353
                  n130 = Dequeue Element(queue=w358, error in (no error)=w359) -> (error out=w357:errorcluster)  [unwired: 1 in, 3 out]
                }
              }
            }
            n131 = property on="Stop" class="Bool"(error in=w342, "DisabledEnum"=T13."Disabled and Grayed Out" ("Disabled")) -> (error out=w343:errorcluster)  [unwired: 1 in, 1 out]
          }
          event User Event {
            n132 = event-data() -> ("MapPointsArray"=w365:cluster{"X":i32, "Y":i32}[], "Laser Point Coor"=w369:cluster{"X":i32, "Y":i32}, "Microscope Image Ref"=w361:T1)  [unwired: 1 in, 4 out]
            n133 = Array Size(array=w365) -> (size(s)=→"Number of Points Selected":i32)
            n134 = To Variant(anything=w365) -> (Variant=w366:variant)
            n135 = To Variant(anything=w369) -> (Variant=w370:variant)
            n136 = To Variant(anything=w361) -> (Variant=w362:variant)
            n137 = call "Microscope Controller GFV.vi"("error in (no error)"=w372, "MicroscopeEnum"=MicroscopeControllerEnum."InsertLaserPoint!", "Data in"=w370) -> ("error out"=w368:errorcluster)  [unwired: 7 in, 1 out]
            n138 = call "Microscope Controller GFV.vi"("error in (no error)"=w368, "MicroscopeEnum"=MicroscopeControllerEnum."InsertMapPoints!", "Data in"=w366) -> ("error out"=w364:errorcluster)  [unwired: 7 in, 1 out]
            n139 = call "Microscope Controller GFV.vi"("error in (no error)"=w364, "MicroscopeEnum"=MicroscopeControllerEnum."InsertMicroscopeImageRef!", "Data in"=w362) -> ("error out"=w360:errorcluster)  [unwired: 7 in, 1 out]
          }
          event "CaptureMicroscopeImageButton": Value Change {
            w387 = T15 4 items=["Grayscale (U8)", "Grayscale (I16)", "Grayscale (SGL)", "Complex (CSG)", "RGB (U32)", "HSL (U32)", "RGB (U64)", "Grayscale (U16)"] ("Image Type")
            n140 = event-data() -> ()  [unwired: 1 in, 6 out]
            n141 = call "Microscope Controller GFV.vi"("error in (no error)"=w393, "MicroscopeEnum"=MicroscopeControllerEnum."GetMicroscopeImageRef") -> ("error out"=w392:errorcluster, "Data Out"=w391:variant)  [unwired: 8 in]
            n142 = Variant To Data(error in=w392, type=T1 refnum ("Microscope Image Ref"), Variant=w391) -> (data=w384:T1, error out=w386:errorcluster)
            n143 = call "IMAQ Create"("Image Name"="Microscope Image Capture", "Image Type"=w387, "error in (no error)"=w386) -> ("New Image"=w383:T1, "error out"=w385:errorcluster)  [unwired: 1 in, 1 out]
            n144 = call "IMAQ Copy"("error in (no error)"=w385, "Image Dst"=w383, "Image Src"=w384) -> ("error out"=w381:errorcluster, "Image Dst Out"=w380:T1)  [unwired: 3 in]
            "User Picture" <- w380
            n145 = call-poly "IMAQ Write String"("error in (no error)"=w381, "Image Quality"=u32 750, "Image"=w380) -> ("error out"=w378:errorcluster, "FileString"=w377:string)  [unwired: 6 in, 1 out]
            n146 = To Variant(anything=w377) -> (Variant=w379:variant)
            n147 = call "MapScriptActorGFV.vi"("error in (no error)"=w378, "MapScriptEnum"=MapScriptGFVEnum."InsertMicroscopeImage", "Data in"=w379) -> ("error out"=w375:errorcluster)  [unwired: 7 in, 1 out]
          }
          event "Reset Measurement": Value Change {
            w414 = T15 4 items=["Grayscale (U8)", "Grayscale (I16)", "Grayscale (SGL)", "Complex (CSG)", "RGB (U32)", "HSL (U32)", "RGB (U64)", "Grayscale (U16)"] ("Image Type")
            n148 = event-data() -> ()  [unwired: 1 in, 6 out]
            n149 = property on="Experiment Title" class="Str"(error in=w417, "Val(Sgnl)"="" ("Experiment Title")) -> (error out=w397:errorcluster)  [unwired: 1 in, 1 out]
            n150 = To Variant(anything="" ("Image Name")) -> (Variant=w399:variant)
            n151 = call "MapScriptActorGFV.vi"("error in (no error)"=w397, "MapScriptEnum"=MapScriptGFVEnum."InsertMicroscopeImage", "Data in"=w399) -> ("error out"=w396:errorcluster)  [unwired: 7 in, 1 out]
            n152 = call "IMAQ Create"("Image Name"="Microscope Image Capture", "Image Type"=w414, "error in (no error)"=w396) -> ("New Image"=w411:T1, "error out"=w412:errorcluster)  [unwired: 1 in, 1 out]
            n153 = property on="User Picture" class="ImageControl"(error in=w412, "Value"=w411) -> (error out=w403:errorcluster)  [unwired: 1 in, 1 out]
            n154 = call "DatabaseControllerGFV.vi"("error in (no error)"=w403, "Enum"=DatabaseContollerGFVenum."Get Experiment Number!") -> ("error out"=w407:errorcluster, "Data Out"=w406:variant)  [unwired: 8 in]
            n155 = Variant To Data(error in=w407, type=1, Variant=w406) -> (data=w402:i32, error out=w408:errorcluster)
            n156 = To Variant(anything=w402) -> (Variant=w410:variant)
            n157 = call "MapScriptActorGFV.vi"("error in (no error)"=w408, "MapScriptEnum"=MapScriptGFVEnum."InsertExperimentNumber", "Data in"=w410) -> ("error out"=w401:errorcluster)  [unwired: 7 in, 1 out]
            n158 = property on="Experiment No." class="DigNum (strict)"(error in=w401, "Value"=w402) -> (error out=w400:errorcluster)  [unwired: 1 in, 1 out]
          }
          event "Sample Type": Value Change {
            n159 = event-data() -> ("NewVal"=w421:u16)  [unwired: 1 in, 5 out]
            n160 = To Variant(anything="SELECT idsample_type FROM ramanmeas.sample_type WHERE Active=1;") -> (Variant=w431:variant)
            n161 = call "DatabaseControllerGFV.vi"("error in (no error)"=w419, "Enum"=DatabaseContollerGFVenum."GetListOfIndices", "Data in"=w431) -> ("error out"=w428:errorcluster, "Data Out"=w427:variant)  [unwired: 7 in]
            n162 = Variant To Data(error in=w428, type=i32[] [], Variant=w427) -> (data=w425:i32[], error out=w420:errorcluster)
            n163 = Index Array(array=w425, index=w421) -> (element=w423:i32)
            n164 = To Variant(anything=w423) -> (Variant=w422:variant)
            n165 = call "MapScriptActorGFV.vi"("error in (no error)"=w420, "MapScriptEnum"=MapScriptGFVEnum."InsertSampleType", "Data in"=w422) -> ("error out"=w418:errorcluster)  [unwired: 7 in, 1 out]
          }
          event "Experiment Title": Value Change {
            n166 = event-data() -> ("NewVal"=w435:string)  [unwired: 1 in, 5 out]
            n167 = To Variant(anything=w435) -> (Variant=w436:variant)
            n168 = call "MapScriptActorGFV.vi"("error in (no error)"=w437, "MapScriptEnum"=MapScriptGFVEnum."InsertExperimentTitle", "Data in"=w436) -> ("error out"=w434:errorcluster)  [unwired: 7 in, 1 out]
          }
          event Timeout {
            n169 = event-data() -> ()  [unwired: 1 in, 3 out]
            n170 = Get Queue Status(queue=w444, error in (no error)=w441) -> (error out=w442:errorcluster, # elements in queue=w439:i32)  [unwired: 1 in, 6 out]
            "Measurement points left in queue" <- w439
            n171 = Greater Than 0?(x=w439) -> (x > 0?=w443:bool)
            n172 = case shown="True" w443 {
              tunnel: w442 -> [w447 w452]
              tunnel: [w446 w451] -> w440
              frame False {
                n173 = property on="Stop" class="Bool"(error in=w447, "DisabledEnum"=T13."Disabled and Grayed Out" ("Disabled")) -> (error out=w450:errorcluster)  [unwired: 1 in, 1 out]
                n174 = property on="Run" class="Bool"(error in=w450, "DisabledEnum"=T13."Enabled" ("Disabled")) -> (error out=w446:errorcluster)  [unwired: 1 in, 1 out]
              }
              frame True {
                n175 = property on="Stop" class="Bool"(error in=w452, "DisabledEnum"=T13."Enabled" ("Disabled")) -> (error out=w453:errorcluster)  [unwired: 1 in, 1 out]
                n176 = property on="Run" class="Bool"(error in=w453, "DisabledEnum"=T13."Disabled and Grayed Out" ("Disabled")) -> (error out=w451:errorcluster)  [unwired: 1 in, 1 out]
              }
            }
          }
        }
      }
      n177 = Unregister For Events(event registration refnum=w53, error in=w54) -> (error out=w51:errorcluster)
      n178 = Destroy User Event(user event=w52, error in=w51) -> (error out=w44:errorcluster)
      n179 = Destroy User Event(user event=w43, error in=w44) -> (error out=w38:errorcluster)
      n180 = Release Queue(queue=w40, error in (no error)=w39) -> ()  [unwired: 1 in, 3 out]
    }
    frame Error {
    }
  }
  "error out" <- w1
